vi "core_robust_set_cursor_state.vi"(6 "set/unset (set)":enum16{"set", "unset"}(ring), 8 "error in (no error)":errorcluster, 11 "disable click? (T)":bool=TRUE) -> (0 "error out":errorcluster, 3 "front pannel is closed?":bool)   [LabVIEW 2015]
uses:
  ref_tools/polys/poly_this_vis_ref.vi
  ref_tools/name_of_caller.vi
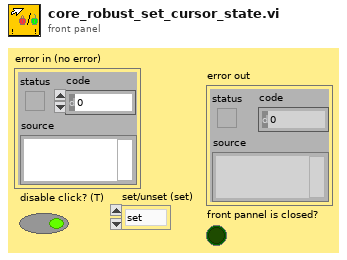
[diagram p1: front panel]
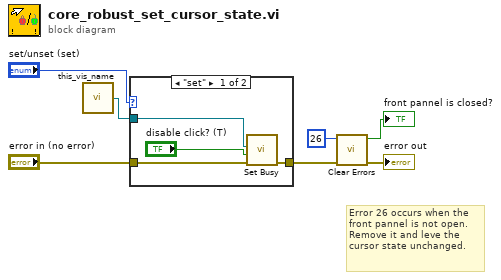
[diagram p0: block diagram]
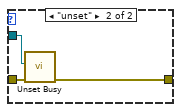
[diagram p2: hidden frame]
diagram:
  # "Error 26 occurs when the front pannel is not open.\nRemove it and leve the cursor state unchanged."
  n1 = call-poly "this_vis_name.vi"() -> ("your ref"=w1:refnum<vi>)  [unwired: 9 in]
  n2 = case shown="\"set\"" "set/unset (set)" {
    tunnel: "error in (no error)" -> [w11 w13]
    tunnel: w1 -> [w10 w14]
    tunnel: [w9 w12] -> w6
    frame "set" {
      n3 = call <vilib>:"Set Busy.vi"("error in (no error)"=w11, "disable click? (T)"="disable click? (T)", "VI reference (current VI)"=w10) -> ("error out"=w9:errorcluster)  [unwired: 7 in, 1 out]
    }
    frame "unset" {
      n4 = call <vilib>:"Unset Busy.vi"("error in (no error)"=w13, "VI reference (current VI)"=w14) -> ("error out"=w12:errorcluster)  [unwired: 9 in]
    }
  }
  n5 = call <vilib>:"Clear Errors.vi"("error in (no error)"=w6, "specific error code to clear (0: all)"=26) -> ("error out"=→"error out":errorcluster, "specific error cleared?"=→"front pannel is closed?":bool)  [unwired: 4 in]
